vi "SetFilterCoeffs.vi"(8 "error in (no error)":errorcluster, 10 "COE file":path, 11 "FPGA ref":T1) -> (0 "error out":errorcluster, 3 "FPGA ref out":T1)   [LabVIEW 2013]
uses:
  controls/settingsFPGAref.ctl
  Utilities/COEfile/CoeFile.lvclass
  FPGA/fpga_settings.ctl
  <vilib>/rvi/interface/common/niFpgaWaitOnOcc.vi
  <vilib>/Utility/error.llb/Error Cluster From Error Code.vi
  <vilib>/rvi/errors/niLvFpgaAdjustHostInterfaceError.vi
  <vilib>/rvi/interface/nirviReadWriteControl/nirviReadWriteControl.xnode
  <vilib>/rvi/interface/nirviMethod/nirviMethod.xnode
  <vilib>/rvi/interface/Simulation/niFpgaSimulationCallBeginRW.vi
  <vilib>/FPGAPlugInAG/Dynamic/niLvFpga_WriteFifo_Dynamic.vi
  <vilib>/rvi/errors/niLvFpgaMergeErrorWithErrorCode.vi
  NiFpgaLv.dll
panel:
  out "shift":i32
  out "Coeffs":fxp<+/-,18,18>[](array[numeric])
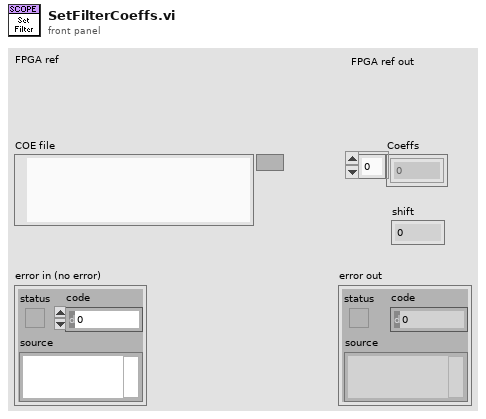
[diagram p1: front panel]
types:
  T1 = typedef "settingsFPGAref.ctl" = refnum<k20>
  T2 = typedef "fpga_settings.ctl" = enum16{"Feedback Enable", "New FIR coeffs", "FIR shift", "Enable filter", "Set Downsample", "Downsample", "CIC Gain", "Record length", "Trigger samples", "Quiet time", "a_am", "b_am", "Use fixed delay", "fixed sin_fi", "fixed cos_fi", "Ki*Tau", "Kp", "Kd_Tau", "Fi_start", "Fi_delta", "DC_offs 0", "DC_offs 1", "Ki*Tau am", "Kp am", "Kd_Tau am"}
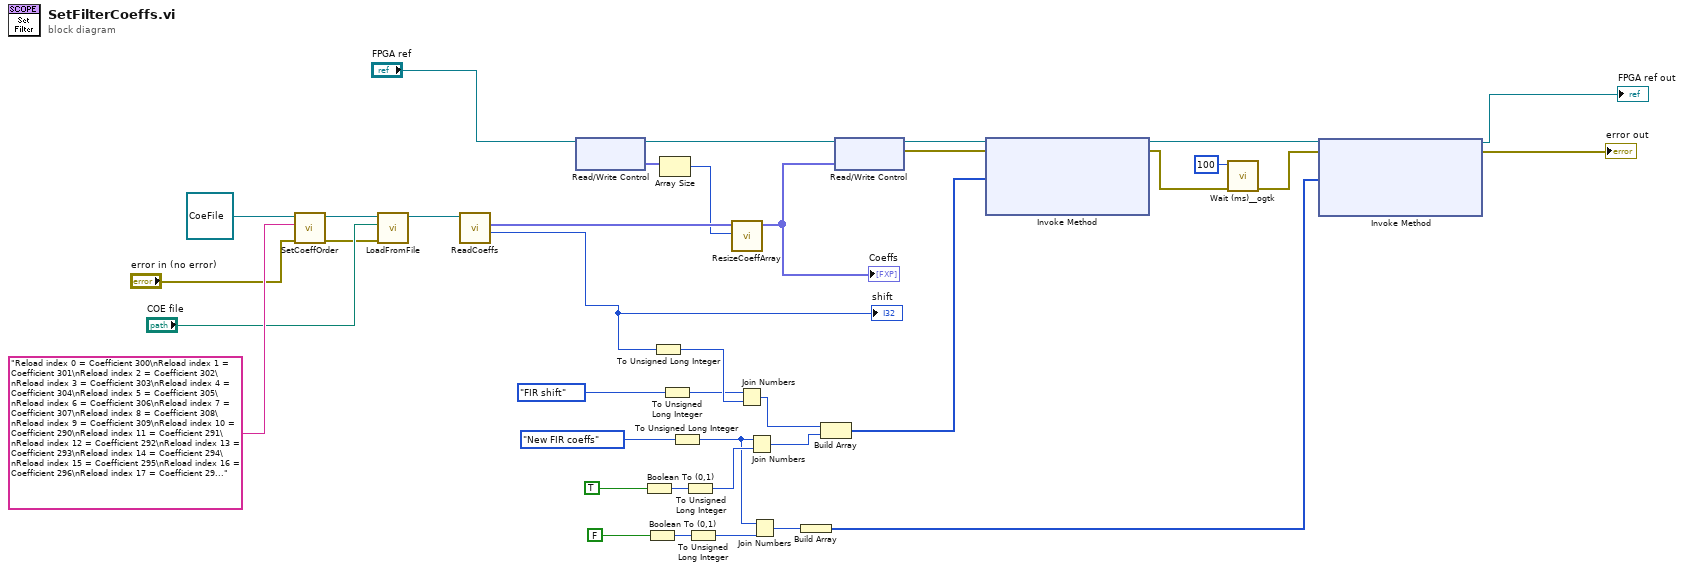
[diagram p0: block diagram]
diagram:
  n1 = call "SetCoeffOrder.vi"("error in (no error)"="error in (no error)", "Order"="Reload index 0 = Coefficient 300\nReload index 1 = Coefficient 301\nReload index 2 = Coefficient 302\nReload index 3 = Coefficient 303\nReload index 4 = Coefficient 304\nReload index 5 = Coefficient 305\nReload index 6 = Coefficient 306\nReload index 7 = Coefficient 307\nReload index 8 = Coefficient 308\nReload index 9 = Coefficient 309\nReload index 10 = Coefficient 290\nReload index 11 = Coefficient 291\nReload index 12 = Coefficient 292\nReload index 13 = Coefficient 293\nReload index 14 = Coefficient 294\nReload index 15 = Coefficient 295\nReload index 16 = Coefficient 296\nReload index 17 = Coefficient 297\nReload index 18 = Coefficient 298\nReload index 19 = Coefficient 299\nReload index 20 = Coefficient 280\nReload index 21 = Coefficient 281\nReload index 22 = Coefficient 282\nReload index 23 = Coefficient 283\nReload index 24 = Coefficient 284\nReload index 25 = Coefficient 285\nReload index 26 = Coefficient 286\nReload index 27 = Coefficient 287\nReload index 28 = Coefficient 288\nReload index 29 = Coefficient 289\nReload index 30 = Coefficient 270\nReload index 31 = Coefficient 271\nReload index 32 = Coefficient 272\nReload index 33 = Coefficient 273\nReload index 34 = Coefficient 274\nReload index 35 = Coefficient 275\nReload index 36 = Coefficient 276\nReload index 37 = Coefficient 277\nReload index 38 = Coefficient 278\nReload index 39 = Coefficient 279\nReload index 40 = Coefficient 260\nReload index 41 = Coefficient 261\nReload index 42 = Coefficient 262\nReload index 43 = Coefficient 263\nReload index 44 = Coefficient 264\nReload index 45 = Coefficient 265\nReload index 46 = Coefficient 266\nReload index 47 = Coefficient 267\nReload index 48 = Coefficient 268\nReload index 49 = Coefficient 269\nReload index 50 = Coefficient 250\nReload index 51 = Coefficient 251\nReload index 52 = Coefficient 252\nReload index 53 = Coefficient 253\nReload index 54 = Coefficient 254\nReload index 55 = Coefficient 255\nReload index 56 = Coefficient 256\nReload index 57 = Coefficient 257\nReload index 58 = Coefficient 258\nReload index 59 = Coefficient 259\nReload index 60 = Coefficient 240\nReload index 61 = Coefficient 241\nReload index 62 = Coefficient 242\nReload index 63 = Coefficient 243\nReload index 64 = Coefficient 244\nReload index 65 = Coefficient 245\nReload index 66 = Coefficient 246\nReload index 67 = Coefficient 247\nReload index 68 = Coefficient 248\nReload index 69 = Coefficient 249\nReload index 70 = Coefficient 230\nReload index 71 = Coefficient 231\nReload index 72 = Coefficient 232\nReload index 73 = Coefficient 233\nReload index 74 = Coefficient 234\nReload index 75 = Coefficient 235\nReload index 76 = Coefficient 236\nReload index 77 = Coefficient 237\nReload index 78 = Coefficient 238\nReload index 79 = Coefficient 239\nReload index 80 = Coefficient 220\nReload index 81 = Coefficient 221\nReload index 82 = Coefficient 222\nReload index 83 = Coefficient 223\nReload index 84 = Coefficient 224\nReload index 85 = Coefficient 225\nReload index 86 = Coefficient 226\nReload index 87 = Coefficient 227\nReload index 88 = Coefficient 228\nReload index 89 = Coefficient 229\nReload index 90 = Coefficient 210\nReload index 91 = Coefficient 211\nReload index 92 = Coefficient 212\nReload index 93 = Coefficient 213\nReload index 94 = Coefficient 214\nReload index 95 = Coefficient 215\nReload index 96 = Coefficient 216\nReload index 97 = Coefficient 217\nReload index 98 = Coefficient 218\nReload index 99 = Coefficient 219\nReload index 100 = Coefficient 200\nReload index 101 = Coefficient 201\nReload index 102 = Coefficient 202\nReload index 103 = Coefficient 203\nReload index 104 = Coefficient 204\nReload index 105 = Coefficient 205\nReload index 106 = Coefficient 206\nReload index 107 = Coefficient 207\nReload index 108 = Coefficient 208\nReload index 109 = Coefficient 209\nReload index 110 = Coefficient 190\nReload index 111 = Coefficient 191\nReload index 112 = Coefficient 192\nReload index 113 = Coefficient 193\nReload index 114 = Coefficient 194\nReload index 115 = Coefficient 195\nReload index 116 = Coefficient 196\nReload index 117 = Coefficient 197\nReload index 118 = Coefficient 198\nReload index 119 = Coefficient 199\nReload index 120 = Coefficient 180\nReload index 121 = Coefficient 181\nReload index 122 = Coefficient 182\nReload index 123 = Coefficient 183\nReload index 124 = Coefficient 184\nReload index 125 = Coefficient 185\nReload index 126 = Coefficient 186\nReload index 127 = Coefficient 187\nReload index 128 = Coefficient 188\nReload index 129 = Coefficient 189\nReload index 130 = Coefficient 170\nReload index 131 = Coefficient 171\nReload index 132 = Coefficient 172\nReload index 133 = Coefficient 173\nReload index 134 = Coefficient 174\nReload index 135 = Coefficient 175\nReload index 136 = Coefficient 176\nReload index 137 = Coefficient 177\nReload index 138 = Coefficient 178\nReload index 139 = Coefficient 179\nReload index 140 = Coefficient 160\nReload index 141 = Coefficient 161\nReload index 142 = Coefficient 162\nReload index 143 = Coefficient 163\nReload index 144 = Coefficient 164\nReload index 145 = Coefficient 165\nReload index 146 = Coefficient 166\nReload index 147 = Coefficient 167\nReload index 148 = Coefficient 168\nReload index 149 = Coefficient 169\nReload index 150 = Coefficient 150\nReload index 151 = Coefficient 151\nReload index 152 = Coefficient 152\nReload index 153 = Coefficient 153\nReload index 154 = Coefficient 154\nReload index 155 = Coefficient 155\nReload index 156 = Coefficient 156\nReload index 157 = Coefficient 157\nReload index 158 = Coefficient 158\nReload index 159 = Coefficient 159\nReload index 160 = Coefficient 140\nReload index 161 = Coefficient 141\nReload index 162 = Coefficient 142\nReload index 163 = Coefficient 143\nReload index 164 = Coefficient 144\nReload index 165 = Coefficient 145\nReload index 166 = Coefficient 146\nReload index 167 = Coefficient 147\nReload index 168 = Coefficient 148\nReload index 169 = Coefficient 149\nReload index 170 = Coefficient 130\nReload index 171 = Coefficient 131\nReload index 172 = Coefficient 132\nReload index 173 = Coefficient 133\nReload index 174 = Coefficient 134\nReload index 175 = Coefficient 135\nReload index 176 = Coefficient 136\nReload index 177 = Coefficient 137\nReload index 178 = Coefficient 138\nReload index 179 = Coefficient 139\nReload index 180 = Coefficient 120\nReload index 181 = Coefficient 121\nReload index 182 = Coefficient 122\nReload index 183 = Coefficient 123\nReload index 184 = Coefficient 124\nReload index 185 = Coefficient 125\nReload index 186 = Coefficient 126\nReload index 187 = Coefficient 127\nReload index 188 = Coefficient 128\nReload index 189 = Coefficient 129\nReload index 190 = Coefficient 110\nReload index 191 = Coefficient 111\nReload index 192 = Coefficient 112\nReload index 193 = Coefficient 113\nReload index 194 = Coefficient 114\nReload index 195 = Coefficient 115\nReload index 196 = Coefficient 116\nReload index 197 = Coefficient 117\nReload index 198 = Coefficient 118\nReload index 199 = Coefficient 119\nReload index 200 = Coefficient 100\nReload index 201 = Coefficient 101\nReload index 202 = Coefficient 102\nReload index 203 = Coefficient 103\nReload index 204 = Coefficient 104\nReload index 205 = Coefficient 105\nReload index 206 = Coefficient 106\nReload index 207 = Coefficient 107\nReload index 208 = Coefficient 108\nReload index 209 = Coefficient 109\nReload index 210 = Coefficient 90\nReload index 211 = Coefficient 91\nReload index 212 = Coefficient 92\nReload index 213 = Coefficient 93\nReload index 214 = Coefficient 94\nReload index 215 = Coefficient 95\nReload index 216 = Coefficient 96\nReload index 217 = Coefficient 97\nReload index 218 = Coefficient 98\nReload index 219 = Coefficient 99\nReload index 220 = Coefficient 80\nReload index 221 = Coefficient 81\nReload index 222 = Coefficient 82\nReload index 223 = Coefficient 83\nReload index 224 = Coefficient 84\nReload index 225 = Coefficient 85\nReload index 226 = Coefficient 86\nReload index 227 = Coefficient 87\nReload index 228 = Coefficient 88\nReload index 229 = Coefficient 89\nReload index 230 = Coefficient 70\nReload index 231 = Coefficient 71\nReload index 232 = Coefficient 72\nReload index 233 = Coefficient 73\nReload index 234 = Coefficient 74\nReload index 235 = Coefficient 75\nReload index 236 = Coefficient 76\nReload index 237 = Coefficient 77\nReload index 238 = Coefficient 78\nReload index 239 = Coefficient 79\nReload index 240 = Coefficient 60\nReload index 241 = Coefficient 61\nReload index 242 = Coefficient 62\nReload index 243 = Coefficient 63\nReload index 244 = Coefficient 64\nReload index 245 = Coefficient 65\nReload index 246 = Coefficient 66\nReload index 247 = Coefficient 67\nReload index 248 = Coefficient 68\nReload index 249 = Coefficient 69\nReload index 250 = Coefficient 50\nReload index 251 = Coefficient 51\nReload index 252 = Coefficient 52\nReload index 253 = Coefficient 53\nReload index 254 = Coefficient 54\nReload index 255 = Coefficient 55\nReload index 256 = Coefficient 56\nReload index 257 = Coefficient 57\nReload index 258 = Coefficient 58\nReload index 259 = Coefficient 59\nReload index 260 = Coefficient 40\nReload index 261 = Coefficient 41\nReload index 262 = Coefficient 42\nReload index 263 = Coefficient 43\nReload index 264 = Coefficient 44\nReload index 265 = Coefficient 45\nReload index 266 = Coefficient 46\nReload index 267 = Coefficient 47\nReload index 268 = Coefficient 48\nReload index 269 = Coefficient 49\nReload index 270 = Coefficient 30\nReload index 271 = Coefficient 31\nReload index 272 = Coefficient 32\nReload index 273 = Coefficient 33\nReload index 274 = Coefficient 34\nReload index 275 = Coefficient 35\nReload index 276 = Coefficient 36\nReload index 277 = Coefficient 37\nReload index 278 = Coefficient 38\nReload index 279 = Coefficient 39\nReload index 280 = Coefficient 20\nReload index 281 = Coefficient 21\nReload index 282 = Coefficient 22\nReload index 283 = Coefficient 23\nReload index 284 = Coefficient 24\nReload index 285 = Coefficient 25\nReload index 286 = Coefficient 26\nReload index 287 = Coefficient 27\nReload index 288 = Coefficient 28\nReload index 289 = Coefficient 29\nReload index 290 = Coefficient 10\nReload index 291 = Coefficient 11\nReload index 292 = Coefficient 12\nReload index 293 = Coefficient 13\nReload index 294 = Coefficient 14\nReload index 295 = Coefficient 15\nReload index 296 = Coefficient 16\nReload index 297 = Coefficient 17\nReload index 298 = Coefficient 18\nReload index 299 = Coefficient 19\nReload index 300 = Coefficient 0\nReload index 301 = Coefficient 1\nReload index 302 = Coefficient 2\nReload index 303 = Coefficient 3\nReload index 304 = Coefficient 4\nReload index 305 = Coefficient 5\nReload index 306 = Coefficient 6\nReload index 307 = Coefficient 7\nReload index 308 = Coefficient 8\nReload index 309 = Coefficient 9", "CoeFile in"=refnum<class "CoeFile.lvclass"> refnum) -> ("error out"=w33:errorcluster, "CoeFile out"=w37:refnum<class "CoeFile.lvclass">)  [unwired: 7 in]
  n2 = call "LoadFromFile.vi"("error in (no error)"=w33, "path"="COE file", "CoeFile in"=w37) -> ("CoeFile out"=w34:refnum<class "CoeFile.lvclass">)  [unwired: 7 in, 1 out]
  n3 = call "ReadCoeffs.vi"("CoeFile in"=w34) -> ("shift"=w6:i32, "Coeffs"=w29:fxp<+/-,18,18>[])  [unwired: 8 in, 1 out]
  "shift" <- w6
  n4 = xnode "Read/Write Control"("FPGA VI Reference In"="FPGA ref") -> ("FPGA VI Reference Out"=w31:T1, "FIR coeffs"=w30:fxp<+/-,18,18>[])  [unwired: 1 in, 1 out]
  n5 = Boolean To (0,1)(Boolean=TRUE ("Set downsample")) -> (0, 1=w16:i16)
  n6 = Boolean To (0,1)(Boolean=FALSE ("Set downsample")) -> (0, 1=w15:i16)
  n7 = To Unsigned Long Integer(number=w6) -> (unsigned 32bit integer=w22:u32)
  n8 = Array Size(array=w30) -> (size(s)=w28:i32)
  n9 = To Unsigned Long Integer(number=fpga_settings."FIR shift" ("FPGA Setting")) -> (unsigned 32bit integer=w21:u32)
  n10 = To Unsigned Long Integer(number=fpga_settings."New FIR coeffs" ("FPGA Setting")) -> (unsigned 32bit integer=w12:u32)
  n11 = To Unsigned Long Integer(number=w16) -> (unsigned 32bit integer=w18:u32)
  n12 = To Unsigned Long Integer(number=w15) -> (unsigned 32bit integer=w13:u32)
  n13 = call "ResizeCoeffArray.vi"("target size"=w28, "Array in"=w29) -> ("Array out"=w27:fxp<+/-,18,18>[])  [unwired: 9 in]
  "Coeffs" <- w27
  n14 = Join Numbers(hi=w21, lo=w22) -> ((hi.lo)=w20:u64)
  n15 = Join Numbers(hi=w12, lo=w18) -> ((hi.lo)=w25:u64)
  n16 = Join Numbers(hi=w12, lo=w13) -> ((hi.lo)=w10:u64)
  n17 = Build Array(w10) -> (w9:u64[])
  n18 = Build Array(w20, w25) -> (w24:u64[])
  n19 = xnode "Read/Write Control"("FPGA VI Reference In"=w31, "FIR coeffs"=w27) -> ("FPGA VI Reference Out"=w4:T1, "error out"=w3:errorcluster)  [unwired: 1 in]
  n20 = xnode "Invoke Method"("FPGA VI Reference In"=w4, "error in"=w3, "Data"=w24) -> ("FPGA VI Reference Out"=w11:T1, "error out"=w8:errorcluster)  [unwired: 1 in, 1 out]
  n21 = call <userlib>:"Wait (ms)__ogtk.vi"("error in (no error)"=w8, "milliseconds to wait"=u32 100) -> ("error out"=w7:errorcluster)  [unwired: 8 in, 1 out]
  n22 = xnode "Invoke Method"("FPGA VI Reference In"=w11, "error in"=w7, "Data"=w9) -> ("FPGA VI Reference Out"=→"FPGA ref out":T1, "error out"=→"error out":errorcluster)  [unwired: 1 in, 1 out]
